vi "Dynamic Dispatching.vi"() -> ()   [LabVIEW 2010]
uses:
  <vilib>/MDSplus/Classes/Tree_Class/Tree.lvclass
  <vilib>/MDSplus/Classes/Data_Class/TreeNode_Class/TreeNode.lvclass
  <vilib>/MDSplus/Classes/Data_Class/Data.lvclass
  <vilib>/MDSplus/Classes/Data_Class/Scalar_Class/Float32_Class/Float32.lvclass
panel:
  in  "SGL in":sgl=5.555
  out "SGL out":sgl
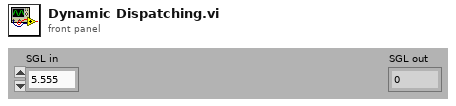
[diagram p1: front panel]
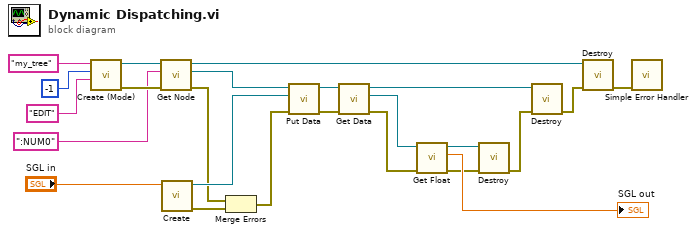
[diagram p0: block diagram]
diagram:
  n1 = call <vilib>:"Create (Mode).vi"("Mode"="EDIT", "Shot"=-1, "Name"="my_tree") -> ("error out"=w20:errorcluster, "Tree out"=w24:refnum<class "Tree.lvclass">)  [unwired: 7 in]
  n2 = call-dynamic "Get Node.vi"("error in (no error)"=w20, "Path"=":NUM0", "Tree in"=w24) -> ("error out"=w12:errorcluster, "Node out"=w18:refnum<class "TreeNode.lvclass">, "Tree out"=w15:refnum<class "Tree.lvclass">)  [unwired: 6 in]
  n3 = call <vilib>:"Create.vi"("SGL in"="SGL in") -> ("error out"=w13:errorcluster, "Float32 out"=w16:refnum<class "Float32.lvclass">)  [unwired: 9 in]
  n4 = Merge Errors(w12, w13) -> (w14:errorcluster)
  n5 = call-dynamic "Put Data.vi"("error in (no error)"=w14, "Data"=w16, "TreeNode in"=w18) -> ("error out"=w10:errorcluster, "TreeNode out"=w11:refnum<class "TreeNode.lvclass">)  [unwired: 7 in]
  n6 = call-dynamic "Get Data.vi"("error in (no error)"=w10, "TreeNode in"=w11) -> ("error out"=w7:errorcluster, "Data out"=w8:refnum<class "Data.lvclass">, "TreeNode out"=w9:refnum<class "TreeNode.lvclass">)  [unwired: 7 in]
  n7 = call-dynamic "Get Float.vi"("error in (no error)"=w7, "Data in"=w8) -> ("error out"=w4:errorcluster, "SGL out"=→"SGL out":sgl, "Data out"=w6:refnum<class "Data.lvclass">)  [unwired: 7 in]
  n8 = call-dynamic "Destroy.vi"("error in (no error)"=w4, "Data in"=w6) -> ("error out"=w3:errorcluster)  [unwired: 9 in]
  n9 = call-dynamic "Destroy.vi"("error in (no error)"=w3, "TreeNode in"=w9) -> ("error out"=w2:errorcluster)  [unwired: 9 in]
  n10 = call-dynamic "Destroy.vi"("error in (no error)"=w2, "Tree in"=w15) -> ("error out"=w1:errorcluster)  [unwired: 9 in]
  n11 = call <vilib>:"Simple Error Handler.vi"("error in (no error)"=w1) -> ()  [unwired: 4 in, 5 out]
